vi "pcb_open_tcp_connection.vi"(8 "error in (no error)":errorcluster) -> (0 "error out":errorcluster, 2 "Welcome msg":string, 3 "TCP Network Connection out":refnum<k5>)   [LabVIEW 2018]
panel:
  out "Numeric":i32
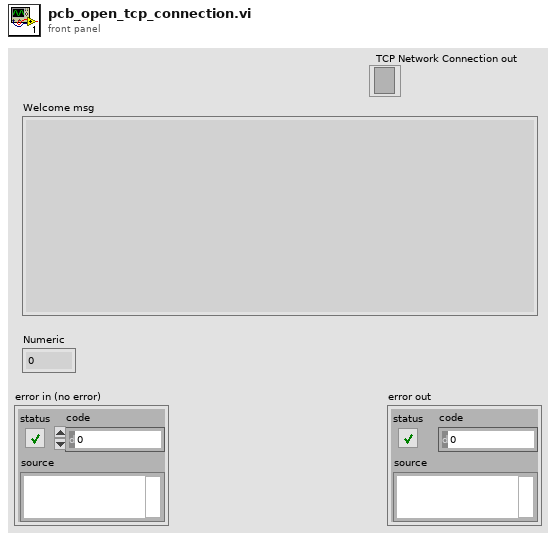
[diagram p1: front panel]
types:
  T1 = enum16{"Standard", "Buffered", "CRLF", "Immediate"}
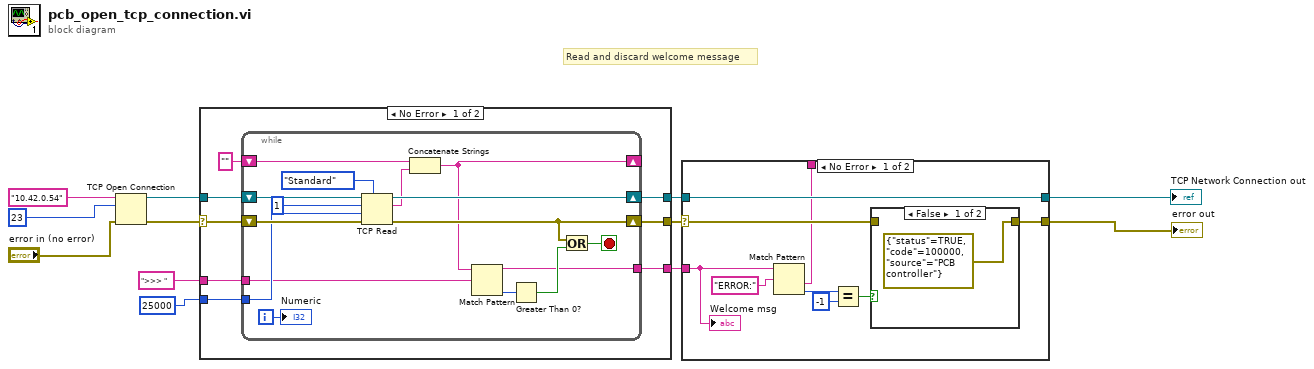
[diagram p0: block diagram]
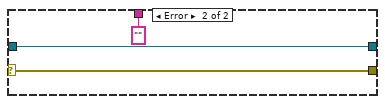
[diagram p3: hidden frame]
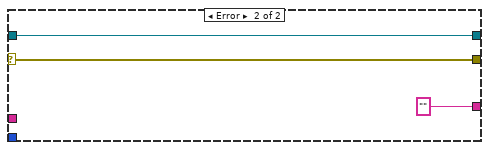
[diagram p4: hidden frame]
diagram:
  # "Read and discard welcome message"
  n1 = TCP Open Connection(address="10.42.0.54" ("IP address"), remote port or service name=u16 23, error in (no error)="error in (no error)") -> (connection ID=w3:refnum<k5>, error out=w1:errorcluster)  [unwired: 2 in]
  n2 = case shown="No Error" w1 {
    selector: w1 -> [w18 w38]
    tunnel: [w20 w39] -> w6
    tunnel: w3 -> [w19 w39]
    tunnel: [w15 w38] -> w7
    tunnel: 25000 ("timeout ms (25000)") -> [w17 _]
    tunnel: ">>> " ("Termination character") -> [w14 _]
    tunnel: [w13 "" ("data out")] -> w8
    frame No Error {
      n3 = while {
        shift-right: [w36] -> w20
        shift-left: w19 -> [w33]
        shift-right: [w26] -> w15
        shift-left: w18 -> [w30]
        shift-right: [w25] -> _
        shift-left: "" -> [w28]
        tunnel: w17 -> [w29]
        tunnel: w14 -> [w24]
        tunnel: [w21] -> w13
        i -> [w35]
        stop <- w27 stop-if-true
        n4 = TCP Read(connection ID=w33, bytes to read=1, error in (no error)=w30, 7:T1."Standard" ("mode (standard)"), 9:w29) -> (connection ID out=w36:refnum<k5>, data out=w34:string, error out=w26:errorcluster)
        n5 = Concatenate Strings(w28, w34) -> (w25:string)
        n6 = Match Pattern(string=w25, regular expression=w24) -> (before substring=w21:string, offset past match=w23:i32)  [unwired: 1 in, 2 out]
        n7 = Greater Than 0?(x=w23) -> (x > 0?=w22:bool)
        n8 = Or(x=w26, y=w22) -> (x .or. y?=w27:bool)
        "Numeric" <- w35
      }
    }
    frame Error {
    }
  }
  n9 = case shown="No Error" w7 {
    selector: w7 -> [w46 w53]
    tunnel: [w47 w53] -> w11
    tunnel: w6 -> [w45 w52]
    tunnel: [w45 w52] -> w10
    tunnel: w8 -> [w41 _]
    tunnel: [w40 "" ("data out")] -> _
    frame No Error {
      n10 = Match Pattern(string=w41, regular expression="ERROR:" ("search string")) -> (after substring=w40:string, offset past match=w42:i32)  [unwired: 1 in, 2 out]
      n11 = Equal?(x=w42, y=-1) -> (x = y?=w44:bool)
      n12 = case shown="False" w44 {
        tunnel: w46 -> [_ w50]
        tunnel: [errorcluster {"status"=TRUE, "code"=100000, "source"="PCB controller"} ("error in (no error) 2") w50] -> w47
        frame False {
        }
        frame True {
        }
      }
      "Welcome msg" <- w41
    }
    frame Error {
    }
  }
  "error out" <- w11
  "TCP Network Connection out" <- w10
